vi "dfd_TF to Lattice AR.vi"(9 "section type":T1(ring), 10 "denominator":dbl[](array[numeric]) format="%.2f", 11 "numerator":dbl[](array[numeric])=[1.0] format="%.2f") -> (0 "fail?":bool, 1 "gain":dbl format="%.2f", 2 "k [1~M]":dbl[](array[numeric]) format="%.2f")   [LabVIEW 2017, in "NI_DigFilterLicensed.lvlib"]
uses:
  <vilib>/addons/Digital Filter Design/NI_DigFilterLicensed.lvlib
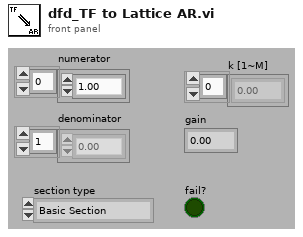
[diagram p1: front panel]
types:
  T1 = enum16{"Basic Section", "One Multiplier Section", "Normalized Section"}
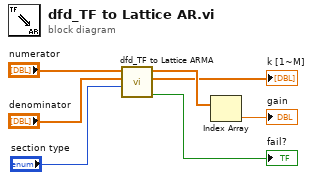
[diagram p0: block diagram]
diagram:
  n1 = call <vilib>:"dfd_TF to Lattice ARMA.vi"("section type"="section type", "denominator"="denominator", "numerator"="numerator") -> ("fail?"=→"fail?":bool, "k [1~M]"=→"k [1~M]":dbl[], "v [0~M]"=w2:dbl[])  [unwired: 6 out]
  n2 = Index Array(array=w2) -> (element=→"gain":dbl)  [unwired: 1 in]
